vi "GVSView Model Message.vi"(8 "nData":i32, 9 "sData":string, 10 "sOption":string, 11 "sMsgData":string) -> (0 "nData_Out":i32, 1 "sData_Out":string, 3 "cView_Out":T1)   [LabVIEW 2013]
uses:
  GVSNew View Global.vi
  SubVI/GVSData View Global.vi
  GVSView Global.vi
panel:
  in  "Resize_Panels":bool
  out "Bar_shadow":bool
  in  "splitter_down_flag":bool=TRUE
  in  "sMsgAction":string
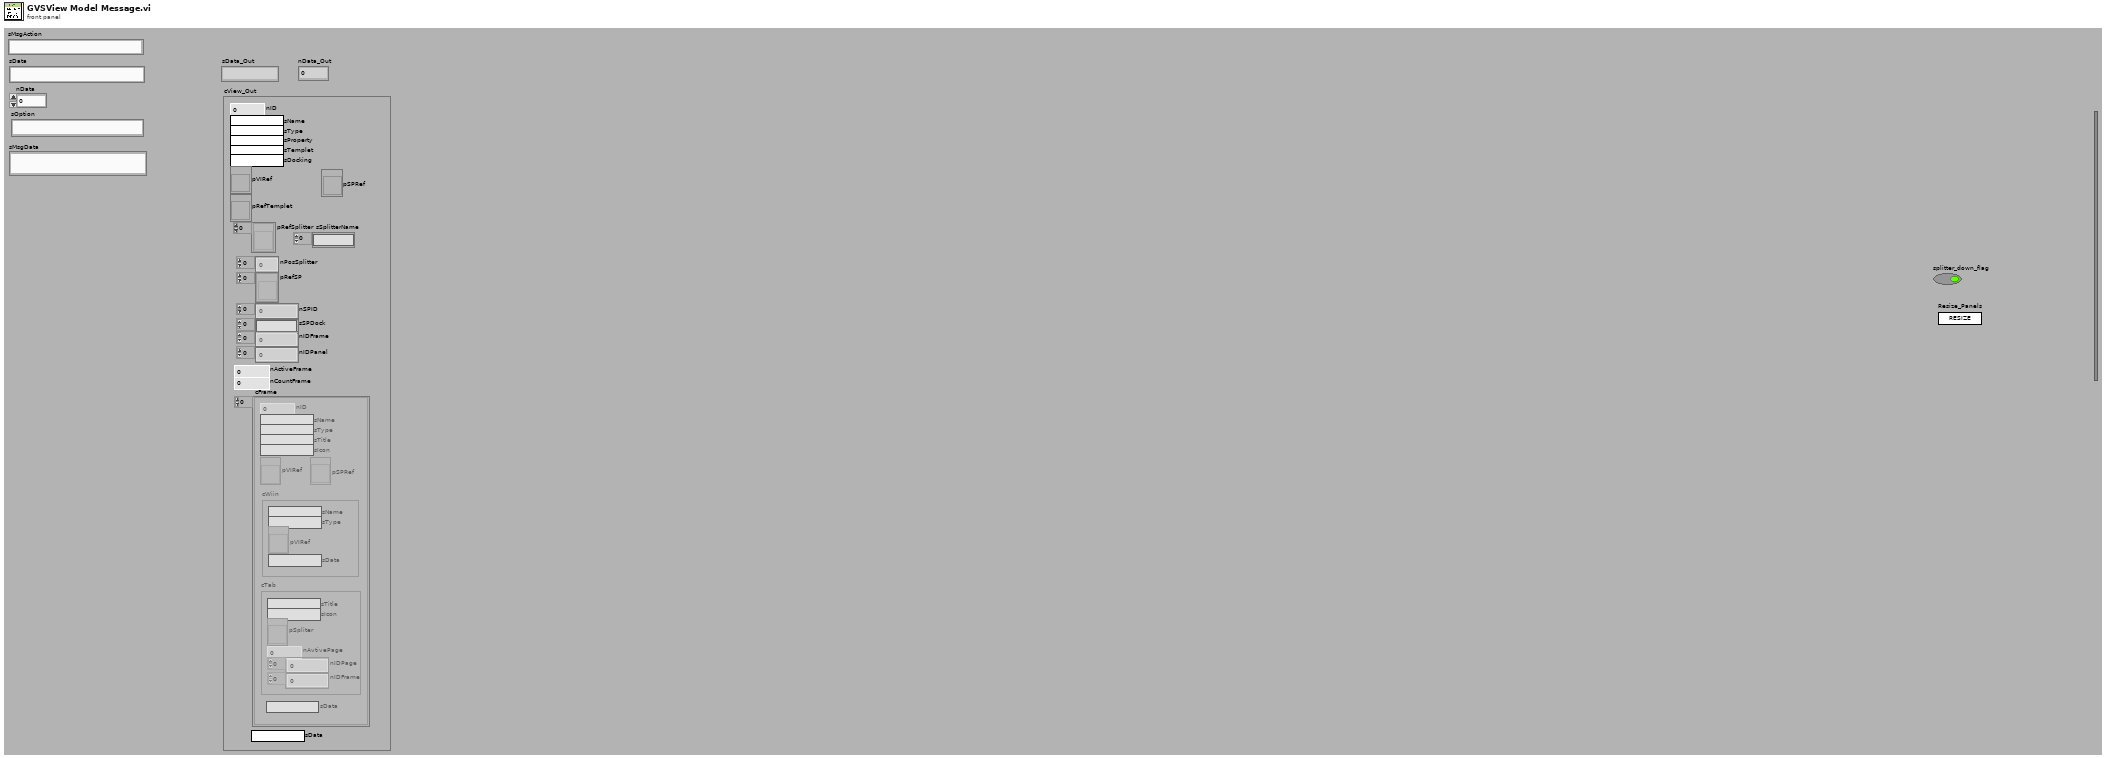
[diagram p1: front panel]
types:
  T1 = cluster{"nID":i32, "sName":string, "sType":string, "sProperty":string, "sTemplet":string, "sDocking":string, "pVIRef":refnum<vi>, "pSPRef":refnum<vi>, "pRefTemplet":refnum<vi>, "pRefSplitter":refnum<vi>[], "nPosSplitter":i32[], "pRefSP":refnum<vi>[], "nSPID":i32[], "sSPDock":string[], "nIDFrame":i32[], "nIDPanel":i32[], "nActiveFrame":i32, "nCountFrame":i32, "cFrame":cluster{"nID":i32, "sName":string, "sType":string, "sTitle":string, "sIcon":string, "pVIRef":refnum<vi>, "pSPRef":refnum<vi>, "cWiin":cluster{"sName":string, "sType":string, "pVIRef":refnum<vi>, "sData":string}, "cTab":cluster{"sTitle":string, "sIcon":string, "pSpliter":refnum<vi>, "nAvtivePage":i32, "nIDPage":i32[], "nIDFrame":i32[]}, "sData":string}[], "sData":string, "sSplitterName":string[]}
  T2 = typedef "Graph Main Info Cluster.ctl" = cluster{"Selected_BarIdx":i32, "Selected_PanelIdx":i32, "Graph Main VIRef":refnum<vi>, "ToolBarClick":bool, "Spliter Ref Array":refnum<vi>[], "Panel Ref Array":refnum<vi>[], "Spliter_matrix":i32[][], "Panel_matrix":i32[][], "child_spliterIdx_matrix":i32[][], "split_pos_matrix":i32[][], "Title State":bool, "sQueueName":string, "Frame nID":i32, "Graph VIRef Array":cluster{"Graph VIRef":refnum<vi>, "Panel Idx":i32, "Frame VIRef":refnum<vi>, "Icon Ring":i32, "Graph Type":string}[], "View Type":string}
  T3 = cluster{"Graph VIRef":refnum<vi>, "Panel Idx":i32, "Frame VIRef":refnum<vi>, "Icon Ring":i32, "Graph Type":string}[]
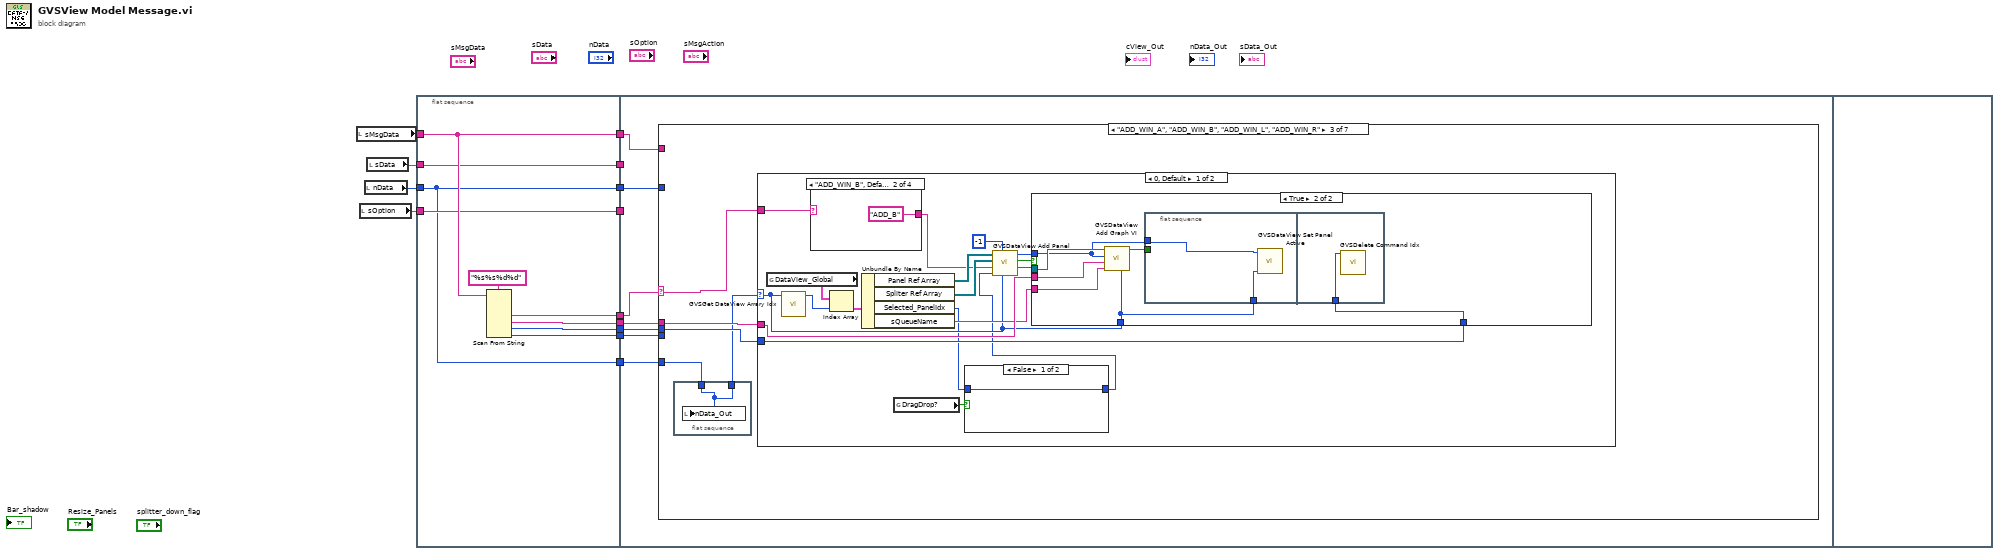
[diagram p0: block diagram]
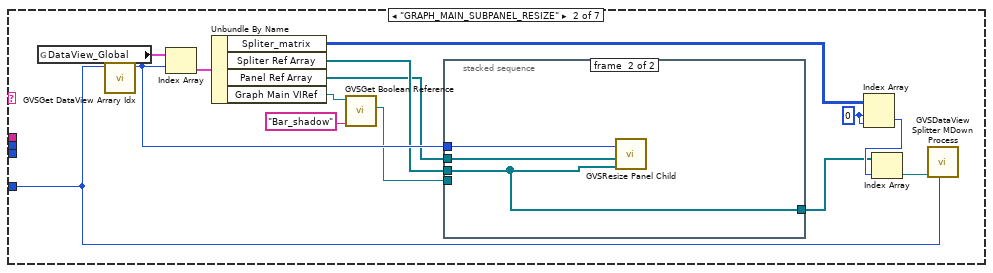
[diagram p3: hidden frame]
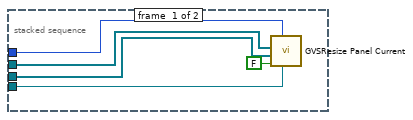
[diagram p4: hidden frame]
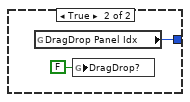
[diagram p5: hidden frame]
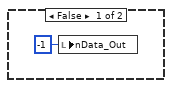
[diagram p6: hidden frame]
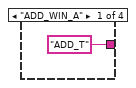
[diagram p7: hidden frame]
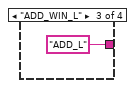
[diagram p8: hidden frame]
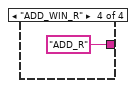
[diagram p9: hidden frame]
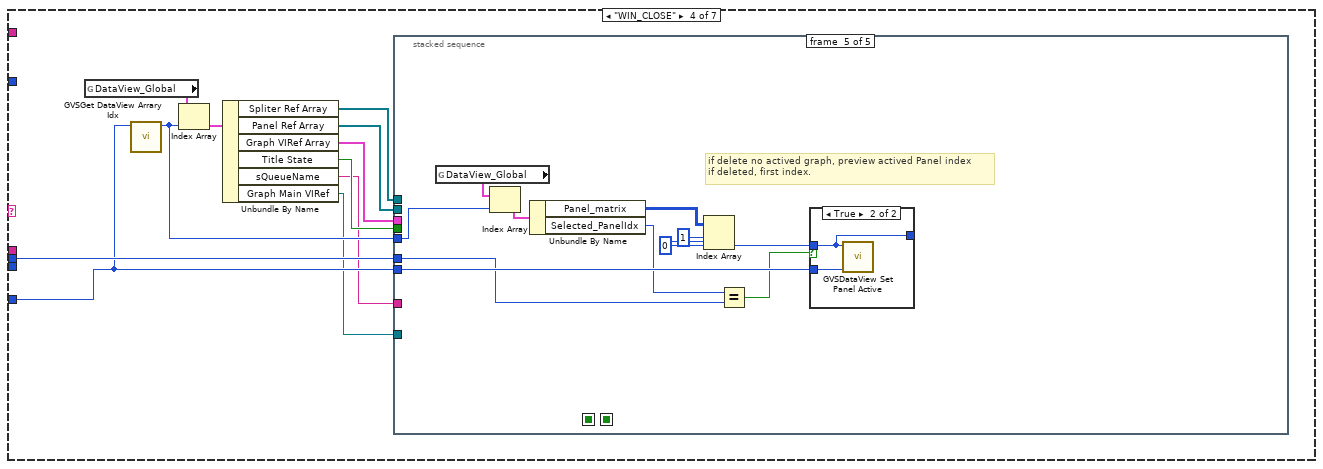
[diagram p11: hidden frame]
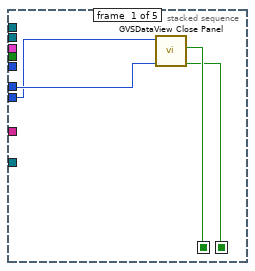
[diagram p12: hidden frame]
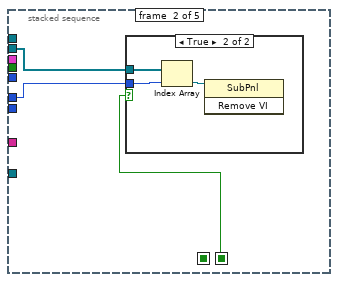
[diagram p13: hidden frame]
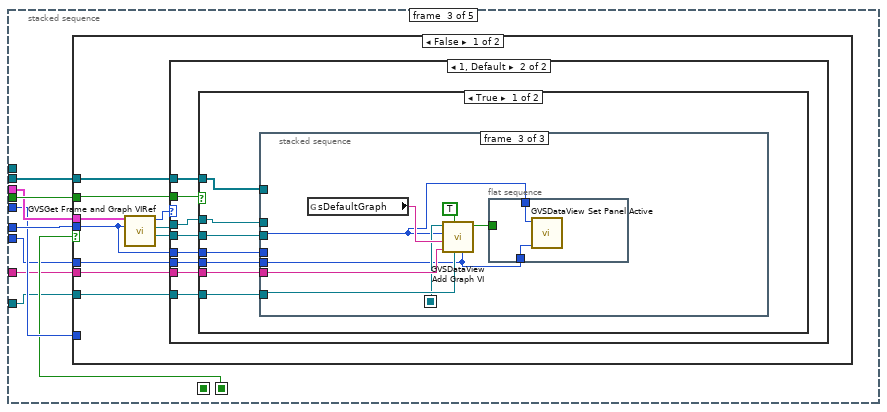
[diagram p15: hidden frame]
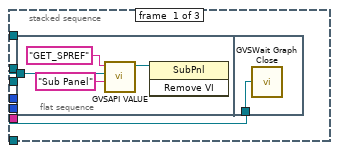
[diagram p17: hidden frame]
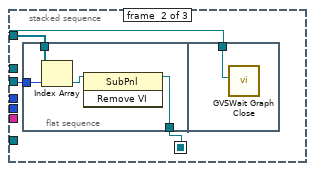
[diagram p18: hidden frame]
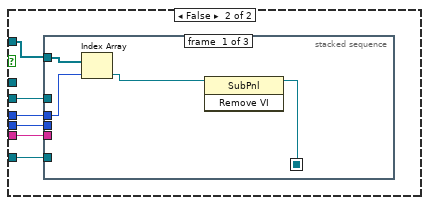
[diagram p19: hidden frame]
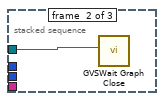
[diagram p20: hidden frame]
diagram:
  n1 = local read "sMsgData"() -> (w13:string)
  n2 = local read "sOption"() -> (w11:string)
  n3 = local read "nData"() -> (w12:i32)
  n4 = local read "sData"() -> (w5:string)
  n5 = flat-sequence {
    tunnel: w13 -> [w21]
    tunnel: w12 -> [w14]
    tunnel: w11 -> [w16]
    tunnel: [w21] -> w10
    tunnel: [w15] -> w9
    tunnel: [w20] -> w8
    tunnel: [w18] -> w7
    tunnel: [w19] -> w6
    tunnel: w5 -> [w17]
    tunnel: [w17] -> w4
    tunnel: [w14] -> w3
    tunnel: [w16] -> w2
    tunnel: [w14] -> w1
    tunnel: w10 -> [w25]
    tunnel: w9 -> [w29]
    tunnel: w8 -> [w28]
    tunnel: w7 -> [w27]
    tunnel: w6 -> [w26]
    tunnel: w4 -> [_]
    tunnel: w3 -> [w24]
    tunnel: w2 -> [_]
    tunnel: w1 -> [w23]
    frame #0 {
      n6 = Scan From String(format string="%s%s%d%d", input string=w21) -> (output 1=w15:string, output 2=w20:string, output 3=w18:i32, output 4=w19:i32)  [unwired: 2 in, 7 out]
    }
    frame #1 {
      n7 = case shown="\"ADD_WIN_A\", \"ADD_WIN_B\", \"ADD_WIN_L\", \"ADD_WIN_R\"" w29 {
        selector: w29 -> [_ _ w55 _ w255 _ _]
        tunnel: w28 -> [_ _ w56 _ _ _ _]
        tunnel: w27 -> [_ _ w54 w104 w256 _ _]
        tunnel: w26 -> [_ _ _ _ _ _ _]
        tunnel: w25 -> [_ _ _ _ _ _ _]
        tunnel: w24 -> [_ _ _ _ _ _ _]
        tunnel: w23 -> [_ w30 w53 w103 w254 _ _]
        frame Default {
        }
        frame "GRAPH_MAIN_SUBPANEL_RESIZE" {
          w41 = 0 ("index (row)")
          n8 = global read "GVSNew View Global.vi" "DataView_Global"() -> (w34:T2[])
          n9 = call "GVSGet DataView Arrary Idx.vi"("DataView Idx In"=w30) -> ("DataView Arrary Idx out"=w43:i32)  [unwired: 10 in]
          n10 = Index Array(array=w34, index=w43) -> (element=w35:T2)
          n11 = Unbundle By Name(w35) -> ("Spliter_matrix"=w39:i32[][], "Spliter Ref Array"=w37:refnum<vi>[], "Panel Ref Array"=w36:refnum<vi>[], "Graph Main VIRef"=w33:refnum<vi>)
          n12 = call "GVSGet Boolean Reference.vi"("Label Name"="Bar_shadow", "VI Refnum"=w33) -> ("Boolean Ref"=w31:refnum<vi>)  [unwired: 7 in, 2 out]
          n13 = stacked-sequence {
            tunnel: w37 -> [w47 w49]
            tunnel: w36 -> [w48 w51]
            tunnel: w43 -> [w46 w50]
            tunnel: [_ w49] -> w38
            tunnel: w31 -> [w45 _]
            frame #0 {
              n14 = call "GVSResize Panel Current.vi"("Bar_shadow"=w45, "DataView Array Idx"=w46, "close_panel"=FALSE, "spliter array"=w47, "SubPanel array"=w48) -> ()  [unwired: 7 in]
            }
            frame #1 {
              n15 = call "GVSResize Panel Child.vi"("spliter array"=w49, "SubPanel array"=w51, "DataView Array Idx"=w50) -> ()  [unwired: 9 in]
            }
          }
          n16 = Index Array(array=w39, index (row)=w41, index (col)=w41) -> (element=w42:i32)
          n17 = Index Array(array=w38, index=w42) -> (element=w40:refnum<vi>)
          n18 = call "GVSDataView Splitter MDown Process.vi"("DataView Index"=w30, "Selected Spliter Ref"=w40) -> ()  [unwired: 9 in, 1 out]
        }
        frame "ADD_WIN_A", "ADD_WIN_B", "ADD_WIN_L", "ADD_WIN_R" {
          n19 = flat-sequence {
            tunnel: w53 -> [w57]
            tunnel: [w57] -> w52
            frame #0 {
              n20 = local write "nData_Out"(w57) -> ()
            }
          }
          n21 = case shown="0, Default" w52 {
            selector: w52 -> [w62 _]
            tunnel: w55 -> [w72 _]
            tunnel: w56 -> [w64 _]
            tunnel: w54 -> [w61 _]
            frame 0, Default {
              n22 = global read "GVSNew View Global.vi" "DataView_Global"() -> (w75:T2[])
              n23 = call "GVSGet DataView Arrary Idx.vi"("DataView Idx In"=w62) -> ("DataView Arrary Idx out"=w74:i32)  [unwired: 10 in]
              n24 = case shown="\"ADD_WIN_B\", Default" w72 {
                tunnel: ["ADD_T" ("input 1") "ADD_B" ("input 1") "ADD_L" ("input 1") "ADD_R" ("input 1")] -> w68
                frame "ADD_WIN_A" {
                }
                frame "ADD_WIN_B", Default {
                }
                frame "ADD_WIN_L" {
                }
                frame "ADD_WIN_R" {
                }
              }
              n25 = Index Array(array=w75, index=w74) -> (element=w73:T2)
              n26 = Unbundle By Name(w73) -> ("Panel Ref Array"=w70:refnum<vi>[], "Spliter Ref Array"=w69:refnum<vi>[], "Selected_PanelIdx"=w59:i32, "sQueueName"=w63:string)
              n27 = global read "GVSData View Global.vi" "DragDrop?"() -> (w60:bool)
              n28 = case shown="False" w60 {
                tunnel: [w76 w77] -> w58
                tunnel: w59 -> [w76 _]
                frame False {
                }
                frame True {
                  n29 = global read "GVSData View Global.vi" "DragDrop Panel Idx"() -> (w77:i32)
                  n30 = global write "GVSData View Global.vi" "DragDrop?"(FALSE ("DragDrop?")) -> ()
                }
              }
              n31 = call "GVSDataView Add Panel.vi"("DataView Index"=w62, "panel_index"=-1, "Selected Panel Idx"=w58, "SAdd_Pos"=w68, "spliter array"=w69, "SubPanel array"=w70) -> ("Panel Ref"=w65:refnum<vi>, "bResult"=w67:bool, "panel_index_out"=w66:i32)  [unwired: 3 in]
              n32 = case shown="True" w67 {
                tunnel: w66 -> [_ w83]
                tunnel: w65 -> [_ w86]
                tunnel: w64 -> [_ w85]
                tunnel: w63 -> [_ w84]
                tunnel: w61 -> [_ w81]
                tunnel: w62 -> [_ w80]
                frame False {
                  n33 = local write "nData_Out"(-1 ("nData_Out")) -> ()
                }
                frame True {
                  n34 = call "GVSDataView Add Graph VI.vi"("DataView Idx"=w80, "Queue Name"=w84, "GraphType"=w85, "panel_index"=w83, "Panel Ref In"=w86) -> ("bResult"=w82:bool)  [unwired: 6 in]
                  n35 = flat-sequence {
                    tunnel: w83 -> [w88]
                    tunnel: w82 -> [_]
                    tunnel: w80 -> [w87]
                    tunnel: w81 -> [w89]
                    frame #0 {
                      n36 = call "GVSDataView Set Panel Active.vi"("DataView Index"=w87, "Selected Panel Idx In"=w88) -> ()  [unwired: 10 in]
                    }
                    frame #1 {
                      n37 = call "GVSDelete Command Idx.vi"("Command Idx In"=w89) -> ()  [unwired: 11 in]
                    }
                  }
                }
              }
            }
            frame -1 {
            }
          }
        }
        frame "WIN_CLOSE" {
          n38 = global read "GVSNew View Global.vi" "DataView_Global"() -> (w102:T2[])
          n39 = call "GVSGet DataView Arrary Idx.vi"("DataView Idx In"=w103) -> ("DataView Arrary Idx out"=w101:i32)  [unwired: 10 in]
          n40 = Index Array(array=w102, index=w101) -> (element=w96:T2)
          n41 = Unbundle By Name(w96) -> ("Spliter Ref Array"=w100:refnum<vi>[], "Panel Ref Array"=w99:refnum<vi>[], "Graph VIRef Array"=w98:T3, "Title State"=w97:bool, "sQueueName"=w95:string, "Graph Main VIRef"=w94:refnum<vi>)
          n42 = stacked-sequence {
            seq-local: [w108 _ _ _ _] -> [_ _ _ w223 _]
            seq-local: [w106 _ _ _ _] -> [_ w111 w119 _ _]
            tunnel: w104 -> [w107 w109 w123 _ w241]
            tunnel: w103 -> [w105 _ w116 _ w249]
            tunnel: w99 -> [_ w110 w115 w224 _]
            tunnel: w100 -> [_ _ _ w225 _]
            tunnel: w101 -> [_ _ w120 w222 w239]
            tunnel: w98 -> [_ _ w121 _ _]
            tunnel: w97 -> [_ _ w122 _ _]
            tunnel: w95 -> [_ _ w118 _ _]
            tunnel: w94 -> [_ _ w117 _ _]
            frame #0 {
              n43 = call "GVSDataView Close Panel.vi"("Panel_Idx"=w107, "DataView Index"=w105) -> ("bResult"=w106:bool, "bHaveChild"=w108:bool)  [unwired: 7 in, 1 out]
            }
            frame #1 {
              n44 = case shown="True" w111 {
                tunnel: w110 -> [_ w114]
                tunnel: w109 -> [_ w113]
                frame False {
                }
                frame True {
                  n45 = Index Array(array=w114, index=w113) -> (element=w112:refnum<vi>)
                  n46 = invoke class="SubPnl" method="Remove VI"(reference=w112) -> ()  [unwired: 2 in, 3 out]
                }
              }
            }
            frame #2 {
              n47 = case shown="False" w119 {
                tunnel: w123 -> [w128 w200]
                tunnel: w122 -> [w133 w199]
                tunnel: w121 -> [w132 w194]
                tunnel: w120 -> [_ w193]
                tunnel: w118 -> [w129 _]
                tunnel: w117 -> [w127 _]
                tunnel: w116 -> [w126 _]
                tunnel: w115 -> [w125 _]
                frame False {
                  n48 = call "GVSGet Frame and Graph VIRef.vi"("Panel Idx"=w128, "Graph VIRef Array"=w132) -> ("Graph VIRef"=w131:refnum<vi>, "Frame VIRef"=w130:refnum<vi>, "Graph VIRef Array Index"=w124:i32)  [unwired: 5 in, 2 out]
                  n49 = case shown="1, Default" w124 {
                    tunnel: w133 -> [_ w141]
                    tunnel: w131 -> [_ w140]
                    tunnel: w130 -> [_ w139]
                    tunnel: w129 -> [_ w138]
                    tunnel: w128 -> [_ w137]
                    tunnel: w127 -> [_ w136]
                    tunnel: w126 -> [_ w135]
                    tunnel: w125 -> [_ w134]
                    frame -1 {
                    }
                    frame 1, Default {
                      n50 = case shown="True" w141 {
                        tunnel: w140 -> [w147 w180]
                        tunnel: w139 -> [w148 _]
                        tunnel: w138 -> [w146 w179]
                        tunnel: w137 -> [w145 w178]
                        tunnel: w136 -> [w144 w177]
                        tunnel: w135 -> [w143 w176]
                        tunnel: w134 -> [w142 w175]
                        frame True {
                          n51 = stacked-sequence {
                            seq-local: [_ w156 _] -> [_ _ w168]
                            tunnel: w148 -> [w150 w157 _]
                            tunnel: w147 -> [w149 _ _]
                            tunnel: w146 -> [_ _ w171]
                            tunnel: w145 -> [_ w158 w165]
                            tunnel: w144 -> [_ _ w170]
                            tunnel: w143 -> [_ _ w166]
                            tunnel: w142 -> [_ w159 _]
                            frame #0 {
                              n52 = flat-sequence {
                                tunnel: w150 -> [w152]
                                tunnel: w149 -> [w155]
                                frame #0 {
                                n53 = call "GVSAPI VALUE.vi"("sControlName"="Sub Panel", "pVIRef"=w152, "sAction"="GET_SPREF") -> ("pSPRef"=w151:refnum<vi>)  [unwired: 2 in, 6 out]
                                n54 = invoke class="SubPnl" method="Remove VI"(reference=w151) -> ()  [unwired: 2 in, 3 out]
                                }
                                frame #1 {
                                n55 = call "GVSWait Graph Close.vi"("vi reference"=w155) -> ()  [unwired: 11 in]
                                }
                              }
                            }
                            frame #1 {
                              n56 = flat-sequence {
                                tunnel: w159 -> [w163]
                                tunnel: w158 -> [w162]
                                tunnel: [w160] -> w156
                                tunnel: w157 -> [w164]
                                frame #0 {
                                n57 = Index Array(array=w163, index=w162) -> (element=w161:refnum<vi>)
                                n58 = invoke class="SubPnl" method="Remove VI"(reference=w161) -> (reference out=w160:refnum<vi>)  [unwired: 2 in, 2 out]
                                }
                                frame #1 {
                                n59 = call "GVSWait Graph Close.vi"("vi reference"=w164) -> ()  [unwired: 11 in]
                                }
                              }
                            }
                            frame #2 {
                              n60 = global read "GVSView Global.vi" "sDefaultGraph"() -> (w172:string)
                              n61 = call "GVSDataView Add Graph VI.vi"("DataView Idx"=w166, "Graph Main VIRef In"=w170, "isFirstPanel"=TRUE, "Queue Name"=w171, "GraphType"=w172, "panel_index"=w165, "Panel Ref In"=w168) -> ("bResult"=w167:bool)  [unwired: 4 in]
                              n62 = flat-sequence {
                                tunnel: w166 -> [w174]
                                tunnel: w167 -> [_]
                                tunnel: w165 -> [w173]
                                frame #0 {
                                n63 = call "GVSDataView Set Panel Active.vi"("DataView Index"=w174, "Selected Panel Idx In"=w173) -> ()  [unwired: 10 in]
                                }
                              }
                            }
                          }
                        }
                        frame False {
                          n64 = stacked-sequence {
                            seq-local: [w184 _ _] -> [_ _ w186]
                            tunnel: w180 -> [_ w185 _]
                            tunnel: w179 -> [_ _ w191]
                            tunnel: w178 -> [w182 _ w190]
                            tunnel: w177 -> [_ _ w189]
                            tunnel: w176 -> [_ _ w187]
                            tunnel: w175 -> [w183 _ _]
                            frame #0 {
                              n65 = Index Array(array=w183, index=w182) -> (element=w181:refnum<vi>)
                              n66 = invoke class="SubPnl" method="Remove VI"(reference=w181) -> (reference out=w184:refnum<vi>)  [unwired: 2 in, 2 out]
                            }
                            frame #1 {
                              n67 = call "GVSWait Graph Close.vi"("vi reference"=w185) -> ()  [unwired: 11 in]
                            }
                            frame #2 {
                              n68 = global read "GVSView Global.vi" "sDefaultGraph"() -> (w192:string)
                              n69 = call "GVSDataView Add Graph VI.vi"("DataView Idx"=w187, "Graph Main VIRef In"=w189, "isFirstPanel"=TRUE, "Queue Name"=w191, "GraphType"=w192, "panel_index"=w190, "Panel Ref In"=w186) -> ()  [unwired: 4 in, 1 out]
                            }
                          }
                        }
                      }
                    }
                  }
                }
                frame True {
                  n70 = call "GVSGet Frame and Graph VIRef.vi"("Panel Idx"=w200, "Graph VIRef Array"=w194) -> ("Graph VIRef"=w196:refnum<vi>, "Frame VIRef"=w197:refnum<vi>, "Graph VIRef Array Index"=w198:i32)  [unwired: 5 in, 2 out]
                  n71 = case shown="True" w199 {
                    tunnel: w198 -> [w209 w213]
                    tunnel: w197 -> [_ w214]
                    tunnel: w196 -> [w210 w215]
                    tunnel: [w209 w213] -> w195
                    frame False {
                      n72 = case shown="0, Default" w209 {
                        tunnel: w210 -> [w211 _]
                        frame 0, Default {
                          n73 = disable-structure shown="Disabled" {
                            disable-tunnel: w211 -> [w212 _]
                            frame Disabled {
                              n74 = call "GVSWindow WAIT CLOSE.vi"("vi reference"=w212) -> ()  [unwired: 11 in]
                            }
                            frame Enabled {
                            }
                          }
                          n75 = call "GVSWait Graph Close.vi"("vi reference"=w211) -> ()  [unwired: 11 in]
                        }
                        frame -1 {
                        }
                      }
                    }
                    frame True {
                      n76 = case shown="0, Default" w213 {
                        tunnel: w215 -> [w217 _]
                        tunnel: w214 -> [w216 _]
                        frame 0, Default {
                          n77 = flat-sequence {
                            tunnel: w217 -> [w218]
                            tunnel: w216 -> [w220]
                            frame #0 {
                              n78 = disable-structure shown="Enabled" {
                                disable-tunnel: w218 -> [w219 _]
                                frame Disabled {
                                n79 = call "GVSWindow WAIT CLOSE.vi"("vi reference"=w219) -> ()  [unwired: 11 in]
                                }
                                frame Enabled {
                                }
                              }
                              n80 = call "GVSWait Graph Close.vi"("vi reference"=w218) -> ()  [unwired: 11 in]
                            }
                            frame #1 {
                              n81 = disable-structure shown="Enabled" {
                                disable-tunnel: w220 -> [w221 _]
                                frame Disabled {
                                n82 = call "GVSWindow WAIT CLOSE.vi"("vi reference"=w221) -> ()  [unwired: 11 in]
                                }
                                frame Enabled {
                                }
                              }
                              n83 = call "GVSWait Graph Close.vi"("vi reference"=w220) -> ()  [unwired: 11 in]
                            }
                          }
                        }
                        frame -1 {
                        }
                      }
                    }
                  }
                  n84 = case shown="0, Default" w195 {
                    selector: w195 -> [w207 _]
                    tunnel: w194 -> [w208 _]
                    tunnel: w193 -> [w202 _]
                    frame 0, Default {
                      n85 = Delete From Array(array=w208, index=w207) -> (array with subset deleted=w206:T3)  [unwired: 1 in, 1 out]
                      n86 = global read "GVSNew View Global.vi" "DataView_Global"() -> (w203:T2[])
                      n87 = Index Array(array=w203, index=w202) -> (element=w201:T2)
                      n88 = Bundle By Name(cluster=w201, "Graph VIRef Array"=w206) -> (w205:T2)
                      n89 = Replace Array Subset(array=w203, new element=w205, index=w202) -> (w204:T2[])
                      n90 = global write "GVSNew View Global.vi" "DataView_Global"(w204) -> ()
                    }
                    frame -1 {
                    }
                  }
                }
              }
            }
            frame #3 {
              n91 = case shown="True" w223 {
                tunnel: w224 -> [_ w228]
                tunnel: w225 -> [_ w227]
                tunnel: w222 -> [_ w226]
                frame False {
                }
                frame True {
                  n92 = flat-sequence {
                    tunnel: w228 -> [w233]
                    tunnel: w227 -> [w232]
                    tunnel: w226 -> [w234]
                    tunnel: [w234] -> w231
                    tunnel: [w233] -> w230
                    tunnel: [w232] -> w229
                    tunnel: w231 -> [w238]
                    tunnel: w230 -> [w237]
                    tunnel: w229 -> [w236]
                    frame #0 {
                      n93 = call "GVSResize Panel Current.vi"("DataView Array Idx"=w234, "close_panel"=TRUE, "spliter array"=w232, "SubPanel array"=w233) -> ()  [unwired: 8 in]
                    }
                    frame #1 {
                      n94 = call "GVSResize Panel Child.vi"("spliter array"=w236, "SubPanel array"=w237, "DataView Array Idx"=w238) -> ()  [unwired: 9 in]
                    }
                  }
                }
              }
            }
            frame #4 {
              # "if delete no actived graph, preview actived Panel index\nif deleted, first index."
              n95 = global read "GVSNew View Global.vi" "DataView_Global"() -> (w248:T2[])
              n96 = Index Array(array=w248, index=w239) -> (element=w247:T2)
              n97 = Unbundle By Name(w247) -> ("Panel_matrix"=w246:i32[][], "Selected_PanelIdx"=w242:i32)
              n98 = Index Array(array=w246, index (row)=1, index (col)=0) -> (element=w243:i32)
              n99 = Equal?(x=w242, y=w241) -> (x = y?=w240:bool)
              n100 = case shown="True" w240 {
                tunnel: w249 -> [_ w252]
                tunnel: w243 -> [w250 w251]
                tunnel: [w250 w251] -> _
                frame False {
                }
                frame True {
                  n101 = call "GVSDataView Set Panel Active.vi"("DataView Index"=w252, "Selected Panel Idx In"=w251) -> ()  [unwired: 10 in]
                }
              }
            }
          }
        }
        frame "WIN_ACTIVE", "WIN_TOOLBAR_CLICKED" {
          n102 = stacked-sequence {
            tunnel: w256 -> [w273]
            tunnel: w254 -> [w272]
            tunnel: [w272] -> w253
            frame #0 {
              n103 = call "GVSDataView Set Panel Active.vi"("DataView Index"=w272, "Selected Panel Idx In"=w273) -> ()  [unwired: 10 in]
              n104 = global write "GVSNew View Global.vi" "DV Virtual_sPos"("" ("DV Virtual_sPos")) -> ()
            }
          }
          n105 = case shown="\"WIN_TOOLBAR_CLICKED\"" w255 {
            tunnel: w253 -> [_ w258]
            frame "False", Default {
            }
            frame "WIN_TOOLBAR_CLICKED" {
              n106 = flat-sequence {
                tunnel: w258 -> [w260]
                tunnel: [w259] -> w257
                tunnel: w257 -> [w270]
                frame #0 {
                  n107 = global read "GVSNew View Global.vi" "DataView_Global"() -> (w263:T2[])
                  n108 = call "GVSGet DataView Arrary Idx.vi"("DataView Idx In"=w260) -> ("DataView Arrary Idx out"=w259:i32)  [unwired: 10 in]
                  n109 = Index Array(array=w263, index=w259) -> (element=w262:T2)
                  n110 = Bundle By Name(cluster=w262, "ToolBarClick"=TRUE) -> (w264:T2)
                  n111 = Replace Array Subset(array=w263, new element=w264, index=w259) -> (w261:T2[])
                  n112 = global write "GVSNew View Global.vi" "DataView_Global"(w261) -> ()
                }
                frame #1 {
                  n113 = global read "GVSNew View Global.vi" "DataView_Global"() -> (w271:T2[])
                  n114 = Index Array(array=w271, index=w270) -> (element=w269:T2)
                  n115 = Unbundle By Name(w269) -> ("Graph Main VIRef"=w266:refnum<vi>)
                  n116 = call "GVSView Pic Set TF Data.vi"("sAction"="SetSigByVIRef_TRUE", "pVIRef"=w266, "sData"="ToolbarClicked") -> ()  [unwired: 9 in]
                }
              }
            }
          }
        }
        frame "DOCKING" {
        }
        frame "WIN_MOUSE_MOVE" {
        }
      }
    }
    frame #2 {
    }
  }
